vi "FGV_ListFilter.vi"(7 "Set":bool, 8 "error in (no error)":errorcluster caption="错误输入（无错误）", 11 "Filter":T1={"Timestamp"="", "Channel"="", "ID"="", "Type"=-1, "Format"=-1, "CANType"=-1, "Direction"=-1, "Len"="", "Data"=""} {"Format" items=["全部"=-1, "数据帧"=0, "远程帧"=1]; "Type" items=["全部"=-1, "标准帧"=0, "扩展帧"=1]; "Direction" items=["全部"=-1, "Tx"=1, "Rx"=0]; "CANType" items=["全部"=-1, "CAN"=0, "CANFD"=1, "CANFD加速"=2]}) -> (0 "error out":errorcluster caption="错误输出", 3 "Filter out":T1={"Timestamp"="", "Channel"="", "ID"="", "Type"=-1, "Format"=-1, "CANType"=-1, "Direction"=-1, "Len"="", "Data"=""} {"Format" items=["全部"=-1, "数据帧"=0, "远程帧"=1]; "Type" items=["全部"=-1, "标准帧"=0, "扩展帧"=1]; "Direction" items=["全部"=-1, "Tx"=1, "Rx"=0]; "CANType" items=["全部"=-1, "CAN"=0, "CANFD"=1, "CANFD加速"=2]})   [LabVIEW 2018, in "CAN FD.lvlib"]
uses:
  CAN FD.lvlib
  Typedef/ListFilter.ctl
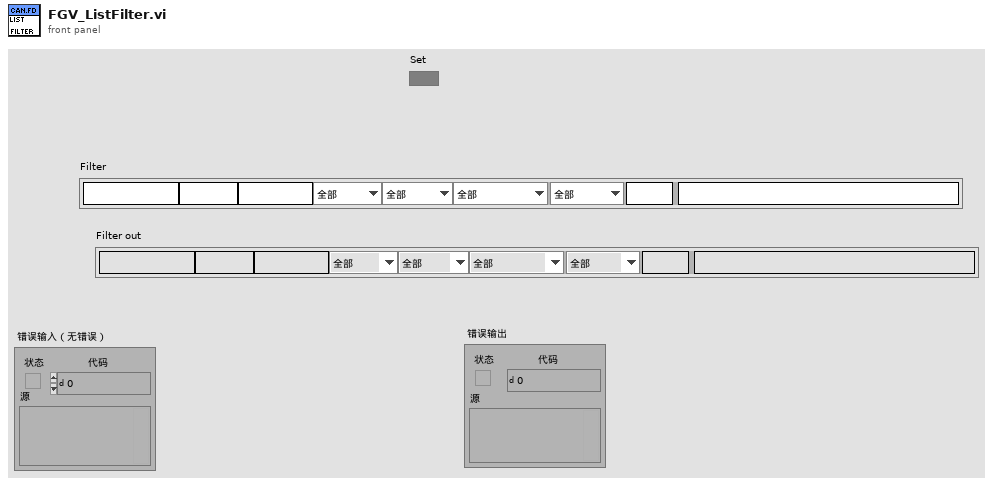
[diagram p1: front panel]
types:
  T1 = typedef "CAN FD.lvlib/ListFilter.ctl" = cluster{"Timestamp":string, "Channel":string, "ID":string, "Type":i16, "Format":i16, "CANType":i16, "Direction":i16, "Len":string, "Data":string}
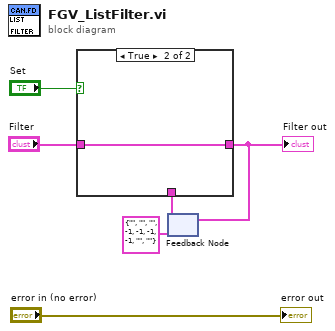
[diagram p0: block diagram]
diagram:
  n1 = feedback #1(T1 {"Timestamp"="", "Channel"="", "ID"="", "Type"=-1, "Format"=-1, "CANType"=-1, "Direction"=-1, "Len"="", "Data"=""} ("Filter")) -> (w2:T1)
  n2 = case shown="True" "Set" {
    tunnel: "Filter" -> [_ w8]
    tunnel: [w7 w8] -> w3
    tunnel: w2 -> [w7 _]
    frame False {
    }
    frame True {
    }
  }
  "Filter out" <- w3
  n3 = feedback-in #1(w3) -> ()
  "error out" <- "error in (no error)"
